vi "FTW-Package-Request-Construct.vi"(8 "error in":errorcluster, 9 "Message":T1, 10 "Frontend Endpoint":refnum<class "FTW-Endpoint.lvclass">) -> (0 "error out":errorcluster, 3 "FTW Incoming Request":refnum<class "FTW-Package-IncomingRequest.lvclass">)   [LabVIEW 2013, in "FTW-Package-IncomingRequest.lvclass"]
uses:
  FTW-Package-IncomingRequest.lvclass
  Message/FTW-Message.ctl
  Endpoint/FTW-Endpoint.lvclass
  FTW-Package-IncomingRequest.lvclass/FTW-Package-IncomingRequest.ctl
panel:
  # "Inputs"
  # "Outputs"
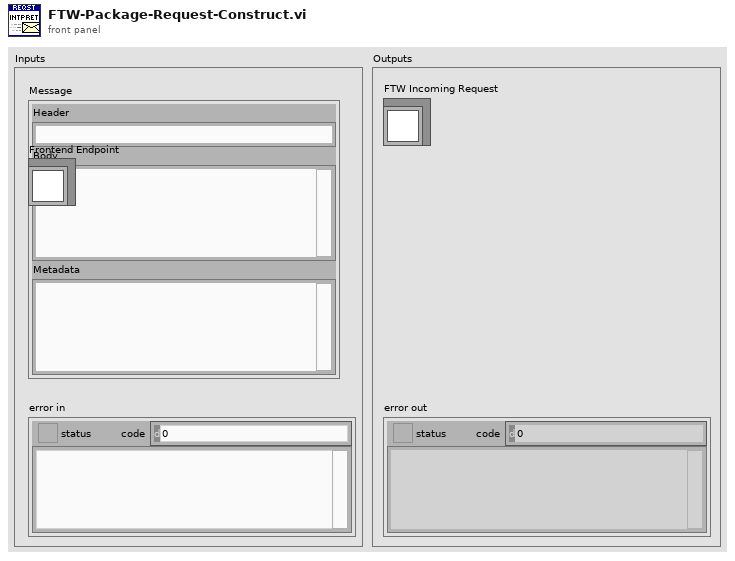
[diagram p1: front panel]
types:
  T1 = typedef "FTW-Message.ctl" = cluster{"Header":string, "Body":string, "Metadata":string}
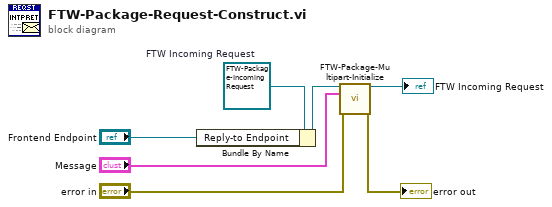
[diagram p0: block diagram]
diagram:
  w3 = refnum<class "FTW-Package-IncomingRequest.lvclass"> refnum  # FTW Incoming Request
  n1 = Bundle By Name(cluster=w3, "Reply-to Endpoint"="Frontend Endpoint") -> (w2:refnum<class "FTW-Package-IncomingRequest.lvclass">)
  n2 = call-dynamic "FTW-Package-Multipart-Initialize.vi"("FTW Message"=w2, "Message"="Message", "error in"="error in") -> ("FTW Message out"=→"FTW Incoming Request":refnum<class "FTW-Package-IncomingRequest.lvclass">, "error out"=→"error out":errorcluster)  [unwired: 11 in]
